vi "Write VoltageLimit.vi"(8 "error in (no error)":errorcluster, 10 "VoltageLimit":dbl, 11 "RMXPowerSupply in":refnum<class "RMXPowerSupply.lvclass">) -> (0 "error out":errorcluster, 3 "RMXPowerSupply out":refnum<class "RMXPowerSupply.lvclass">)   [LabVIEW 2023, in "RMXPowerSupply.lvclass"]
uses:
  RMXPowerSupply.lvclass
  RMXPowerSupply.lvclass/RMXPowerSupply.ctl
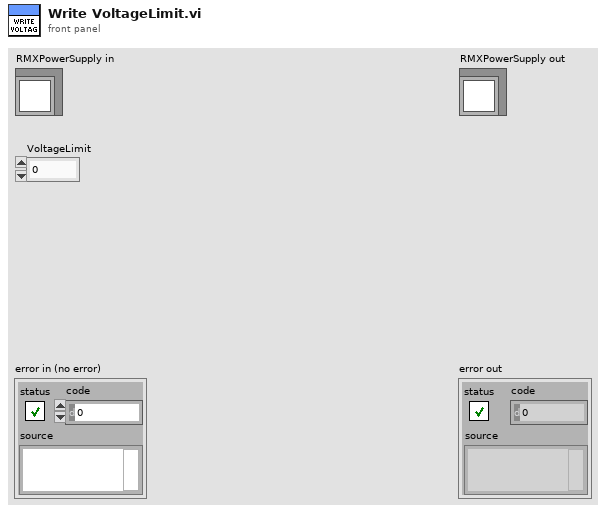
[diagram p1: front panel]
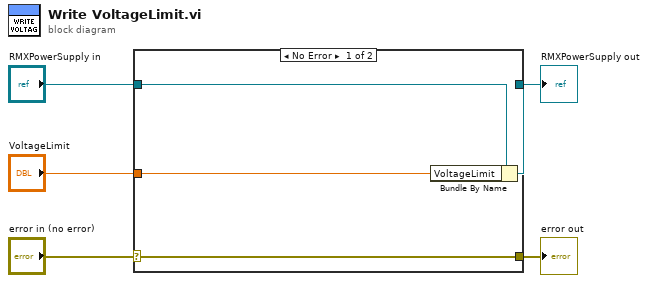
[diagram p0: block diagram]
diagram:
  n1 = case shown="No Error" "error in (no error)" {
    selector: "error in (no error)" -> [w9 w10]
    tunnel: [w9 w10] -> w4
    tunnel: [w7 w11] -> w2
    tunnel: "RMXPowerSupply in" -> [w8 w11]
    tunnel: "VoltageLimit" -> [w6 _]
    frame No Error {
      n2 = Bundle By Name(cluster=w8, "VoltageLimit"=w6) -> (w7:refnum<class "RMXPowerSupply.lvclass">)
    }
    frame Error {
    }
  }
  "error out" <- w4
  "RMXPowerSupply out" <- w2
